vi "ReportHeartbeatPulse.vi"() -> ()   [LabVIEW 2009]
panel:
  in  "Sequence Number (16 bits)":u16=1
  out "Encoded JAUS Message":string
  in  "Command Code":string="B\u0002"
  in  "Destination":T1={"Subsystem Id"=90.0, "Node Id"=1.0, "Component Id"=1.0}
  in  "Source":T1={"Subsystem Id"=3.0, "Node Id"=1.0, "Component Id"=1.0}
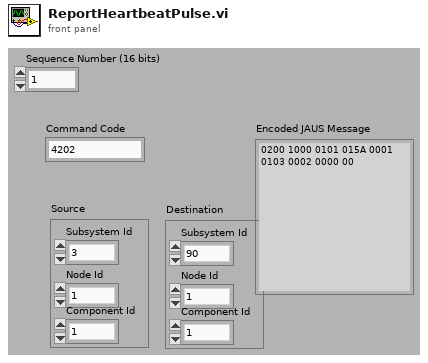
[diagram p1: front panel]
types:
  T1 = cluster{"Subsystem Id":dbl, "Node Id":dbl, "Component Id":dbl}
  T2 = cluster{"unsigned byte array[0]":u8, "unsigned byte array[1]":u8}
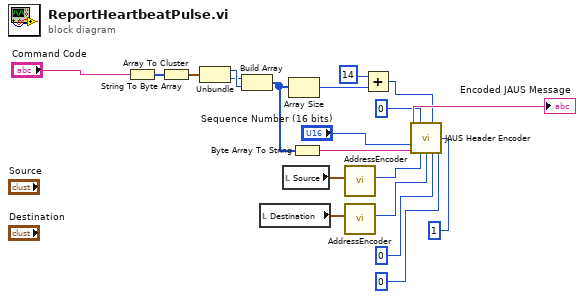
[diagram p0: block diagram]
diagram:
  n1 = String To Byte Array(string="Command Code") -> (unsigned byte array=w5:u8[])
  n2 = Array To Cluster(array=w5) -> (cluster=w4:T2)
  n3 = Unbundle(w4) -> ("unsigned byte array[0]"=w3:u8, "unsigned byte array[1]"=w2:u8)
  n4 = Build Array(w2, w3) -> (w9:u8[])
  n5 = local read "Destination"() -> (w17:T1)
  n6 = local read "Source"() -> (w19:T1)
  n7 = Array Size(array=w9) -> (size(s)=w7:i32)
  n8 = Byte Array To String(unsigned byte array=w9) -> (string=w11:string)
  n9 = call "AddressEncoder.vi"("Address Cluster"=w19) -> ("Address"=w18:u32)  [unwired: 10 in]
  n10 = call "AddressEncoder.vi"("Address Cluster"=w17) -> ("Address"=w16:u32)  [unwired: 10 in]
  n11 = Add(x=14, y=w7) -> (x+y=w6:i32)
  n12 = call "JAUS Header Encoder.vi"("Message Type (0-5)"=u8 0, "Data Size (8-23)"=w6, "Priority(40-41)"=u8 1, "Sequence Number (16 bits)"="Sequence Number (16 bits)", "Payload"=w11, "Source ID (80-95)"=w18, "Destination ID (48-79)"=w16, "Data Flags (46-47)"=u8 0, "Ack/Nak (44-45)"=u8 0) -> ("Encoded JAUS Message"=→"Encoded JAUS Message":string)  [unwired: 6 in]
